vi "Load Sequence Config.vi"(8 "error in (no error)":refnum<class "MultiErrors.lvclass">, 10 "Sequence Config":refnum<class "Sequence Config.lvclass">, 11 "Sequencing in":refnum<class "Sequencing.lvclass">) -> (0 "error out":refnum<class "MultiErrors.lvclass">, 3 "Sequencing out":refnum<class "Sequencing.lvclass">)   [LabVIEW 2020, in "VolatusSeq.lvlib" / "Sequencing.lvclass"]
uses:
  Sequencing.lvclass
  VolatusErrorUtilities/MultiErrors/MultiErrors.lvclass
  C:/dev/lv20CE/relink/lv-volatus/Volatus/Module/Module.lvclass
  VolatusSeqConfig/Sequence Config/Sequence Config.lvclass
  Sequencing.lvclass/Sequencing.ctl
  Volatus/Module/Module.lvclass/Module.ctl
  VolatusErrorUtilities/MultiErrors/MultiErrors.lvclass/MultiErrors.ctl
  VolatusErrorUtilities/MultiErrors/Last Error to Wire.vi
  Sequence/Sequence.lvclass
  Volatus/Module/Module.lvclass
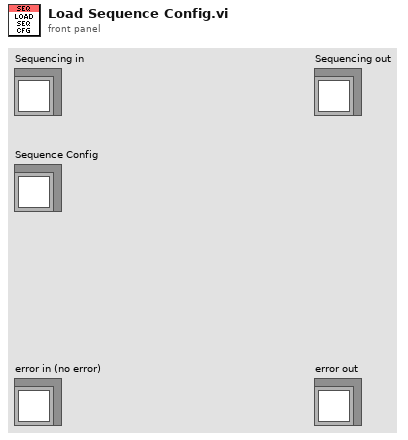
[diagram p1: front panel]
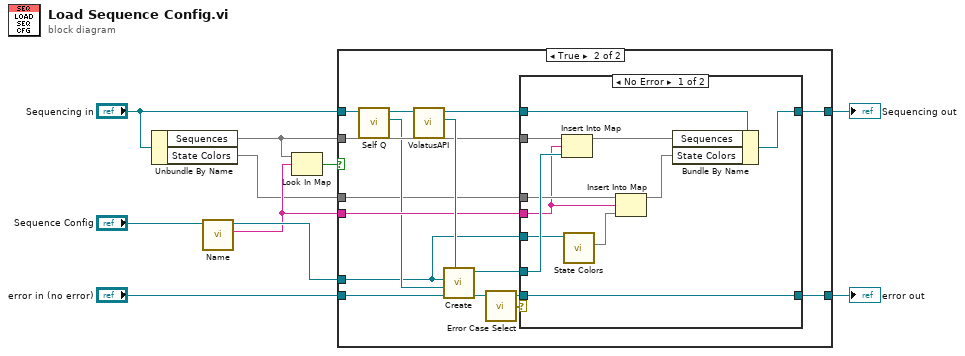
[diagram p0: block diagram]
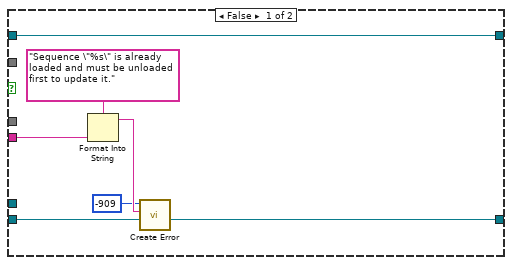
[diagram p2: hidden frame]
diagram:
  n1 = Unbundle By Name("Sequencing in") -> ("Sequences"=w6:map{string, refnum<class "Sequence.lvclass">}, "State Colors"=w3:map{string, map{string, string}})
  n2 = call "Name.vi"("Sequence Config in"="Sequence Config") -> ("Name"=w4:string, "Sequence Config out"=w7:refnum<class "Sequence Config.lvclass">)  [unwired: 8 in, 1 out]
  n3 = Look In Map(map=w6, key=w4) -> (key not found?=w5:bool)  [unwired: 1 in, 1 out]
  n4 = case shown="True" w5 {
    tunnel: [w17 w30] -> w10
    tunnel: "Sequencing in" -> [w17 w29]
    tunnel: w7 -> [_ w23]
    tunnel: w6 -> [_ w28]
    tunnel: w4 -> [w16 w27]
    tunnel: [w11 w26] -> w1
    tunnel: w3 -> [_ w22]
    tunnel: "error in (no error)" -> [w12 w21]
    frame False {
      n5 = Format Into String(format string="Sequence \"%s\" is already loaded and must be unloaded first to update it.", w16) -> (resulting string=w14:string)  [unwired: 2 in, 1 out]
      n6 = call "Create Error.vi"("MultiErrors in"=w12, "Message"=w14, "Code"=-909 ("error code (0)")) -> ("MultiErrors out"=w11:refnum<class "MultiErrors.lvclass">)  [unwired: 8 in]
    }
    frame True {
      n7 = call "Self Q.vi"("Module in"=w29) -> ("Self Q"=w24:refnum<class "MessageQ.lvclass">, "Module out"=w25:refnum<class "Sequencing.lvclass">)  [unwired: 9 in]
      n8 = call "VolatusAPI.vi"("Module in"=w25) -> ("VolatusAPI"=w33:refnum<class "VolatusAPI.lvclass">, "Module out"=w31:refnum<class "Sequencing.lvclass">)  [unwired: 9 in]
      n9 = call "Create.vi"("VolatusAPI"=w33, "error in (no error)"=w21, "Sequencer"=w24, "Sequence Config"=w23) -> ("error out"=w20:refnum<class "MultiErrors.lvclass">, "Sequence out"=w32:refnum<class "Sequence.lvclass">)  [unwired: 6 in]
      n10 = call "Error Case Select.vi"("MultiErrors in"=w20) -> ("MultiErrors out"=w18:refnum<class "MultiErrors.lvclass">, "error out"=w19:errorcluster)  [unwired: 7 in]
      n11 = case shown="No Error" w19 {
        tunnel: w32 -> [w43 _]
        tunnel: w31 -> [w42 w46]
        tunnel: [w40 w46] -> w30
        tunnel: w28 -> [w44 _]
        tunnel: w27 -> [w37 _]
        tunnel: [w34 w45] -> w26
        tunnel: w23 -> [w39 _]
        tunnel: w22 -> [w38 _]
        tunnel: w18 -> [w34 w45]
        frame No Error {
          n12 = Insert Into Map(map in=w44, key=w37, value=w43) -> (map out=w41:map{string, refnum<class "Sequence.lvclass">})  [unwired: 2 out]
          n13 = call "State Colors.vi"("Sequence Config in"=w39) -> ("State Colors"=w36:map{string, string})  [unwired: 8 in, 2 out]
          n14 = Insert Into Map(map in=w38, key=w37, value=w36) -> (map out=w35:map{string, map{string, string}})  [unwired: 2 out]
          n15 = Bundle By Name(cluster=w42, "Sequences"=w41, "State Colors"=w35) -> (w40:refnum<class "Sequencing.lvclass">)
        }
        frame Error {
        }
      }
    }
  }
  "error out" <- w1
  "Sequencing out" <- w10
